vi "mod_Error Dialog.vi"(2 "dialog on warnings?":bool, 3 "error in (no error)":errorcluster) -> (7 "Stop?":bool, 9 "error out":errorcluster)   [LabVIEW 2020, in "niAMT.lvlib"]
uses:
  <vilib>/addons/Modulation/niAMT.lvlib
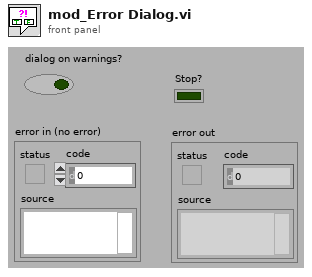
[diagram p1: front panel]
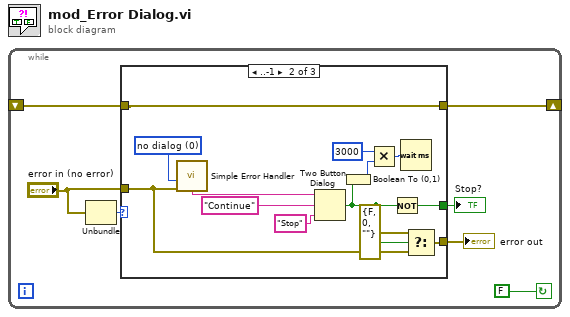
[diagram p0: block diagram]
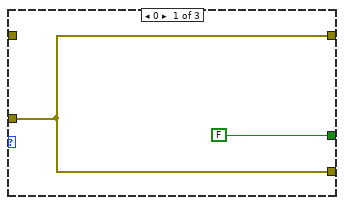
[diagram p2: hidden frame]
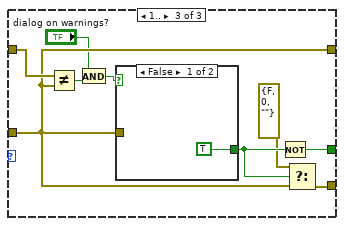
[diagram p3: hidden frame]
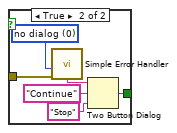
[diagram p4: hidden frame]
diagram:
  n1 = while {
    shift-right: [w2] -> _
    shift-left: _ -> [w1]
    stop <- FALSE continue-if-true
    n2 = Unbundle("error in (no error)") -> ("code"=w6:i32)  [unwired: 2 out]
    n3 = case shown="..-1" w6 {
      tunnel: [FALSE w13 w31] -> w7
      tunnel: "error in (no error)" -> [w8 w12 w25]
      tunnel: [w8 w10 w29] -> w5
      tunnel: [w8 w15 w25] -> w2
      tunnel: w1 -> [_ w15 w26]
      frame 0 {
      }
      frame ..-1 {
        w22 = u16 0 items=["no dialog", "OK message", "continue or stop message"] ("type of dialog (OK msg:1)")
        n4 = call <vilib>:"Simple Error Handler.vi"("type of dialog (OK msg:1)"=w22, "error in (no error)"=w12) -> ("message"=w19:string)  [unwired: 7 out]
        n5 = Two Button Dialog(message=w19, 1:"Stop" ("F button name (\"Cancel\")"), 2:"Continue" ("T button name (\"OK\")")) -> (T button?=w14:bool)
        n6 = Boolean To (0,1)(Boolean=w14) -> (0, 1=w16:i16)
        n7 = Multiply(x=u32 3000 ("milliseconds to wait"), y=w16) -> (x*y=w17:u32)
        n8 = Not(x=w14) -> (.not. x?=w13:bool)
        n9 = Wait (ms)(milliseconds to wait=w17) -> ()  [unwired: 1 out]
        n10 = Select(t=errorcluster {"status"=FALSE, "code"=0, "source"=""}, s=w14, f=w12) -> (s? t:f=w10:errorcluster)
      }
      frame 1.. {
        n11 = Not Equal?(x=w26, y=w25) -> (x != y?=w27:bool)
        n12 = And(x="dialog on warnings?", y=w27) -> (x .and. y?=w24:bool)
        n13 = case shown="False" w24 {
          tunnel: [TRUE ("T button?") w34] -> w30
          tunnel: w25 -> [_ w33]
          frame False {
          }
          frame True {
            w38 = u16 0 items=["no dialog", "OK message", "continue or stop message"] ("type of dialog (OK msg:1)")
            n14 = call <vilib>:"Simple Error Handler.vi"("type of dialog (OK msg:1)"=w38, "error in (no error)"=w33) -> ("message"=w35:string)  [unwired: 7 out]
            n15 = Two Button Dialog(message=w35, 1:"Stop" ("F button name (\"Cancel\")"), 2:"Continue" ("T button name (\"OK\")")) -> (T button?=w34:bool)
          }
        }
        n16 = Not(x=w30) -> (.not. x?=w31:bool)
        n17 = Select(t=errorcluster {"status"=FALSE, "code"=0, "source"=""}, s=w30, f=w25) -> (s? t:f=w29:errorcluster)
      }
    }
    "error out" <- w5
    "Stop?" <- w7
  }
